vi "Module output.vi"   [LabVIEW 2015]
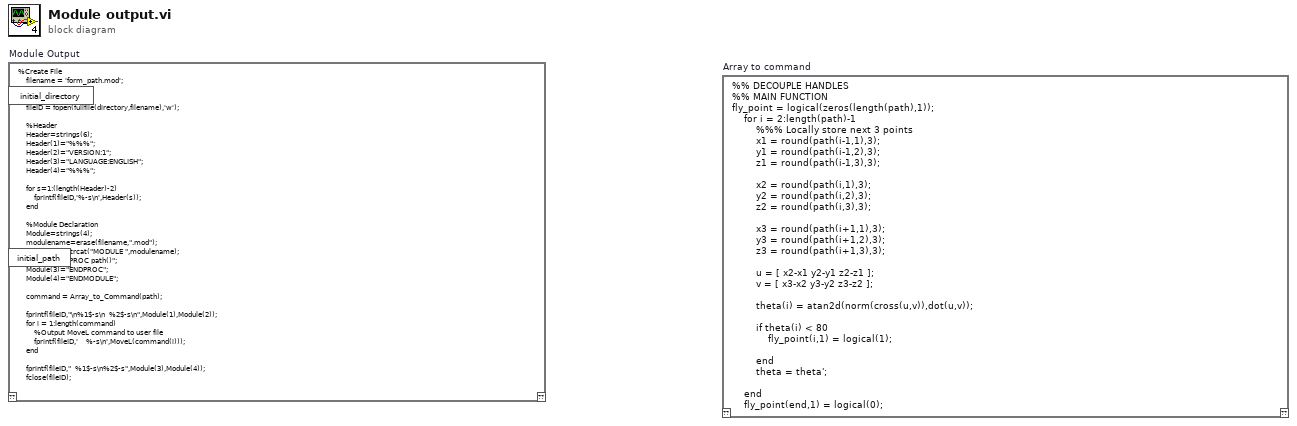
[diagram p0: block diagram]
diagram:
  n1 = script code="%Create File\n    filename = 'form_path.mod';\n   \n    %Open File\n    fileID = fopen(fullfile(directory,filename),'w');\n\n    %Header\n    Header=strings(6);\n    Header(1)=\"%%%\";\n    Header(2)=\"VERSION:1\";\n    Header(3)=\"LANGUAGE:ENGLISH\";\n    Header(4)=\"%%%\";\n    \n    for s=1:(length(Header)-2)\n        fprintf(fileID,'%-s\\n',Header(s));\n    end\n    \n    %Module Declaration\n    Module=strings(4);\n    modulename=erase(filename,\".mod\");\n    Module(1)=strcat(\"MODULE \",modulename);\n    Module(2)=\"PROC path()\";\n    Module(3)=\"ENDPROC\";\n    Module(4)=\"ENDMODULE\";\n    \n    command = Array_to_Command(path);\n    \n    fprintf(fileID,\"\\n%1$-s\\n  %2$-s\\n\",Module(1),Module(2));\n    for i = 1:length(command)\n        %Output MoveL command to user file\n        fprintf(fileID,'    %-s\\n',MoveL(command(i)));\n    end\n        \n    fprintf(fileID,\"  %1$-s\\n%2$-s\",Module(3),Module(4));\n    fclose(fileID);" "Module Output"() -> ()  [unwired: 3 in, 1 out]
  n2 = script code="%% DECOUPLE HANDLES\n%% MAIN FUNCTION\nfly_point = logical(zeros(length(path),1));\n    for i = 2:length(path)-1\n        %%% Locally store next 3 points\n        x1 = round(path(i-1,1),3);\n        y1 = round(path(i-1,2),3);\n        z1 = round(path(i-1,3),3);\n\n        x2 = round(path(i,1),3);\n        y2 = round(path(i,2),3);\n        z2 = round(path(i,3),3);\n\n        x3 = round(path(i+1,1),3);\n        y3 = round(path(i+1,2),3);\n        z3 = round(path(i+1,3),3);\n        \n        u = [ x2-x1 y2-y1 z2-z1 ];\n        v = [ x3-x2 y3-y2 z3-z2 ]; \n        \n        theta(i) = atan2d(norm(cross(u,v)),dot(u,v));\n        \n        if theta(i) < 80\n            fly_point(i,1) = logical(1);\n            \n        end\n        theta = theta';\n\n    end\n    fly_point(end,1) = logical(0);\n    \n    %%% Assign matrix to array of robtargets (command)\n    command = robtarget.empty(length(path),0);\n    for i = 1:length(path)\n        command(i,1).name = ['p',num2str(i)];\n        command(i,1).x = path(i,1);\n        command(i,1).y = path(i,2);\n        command(i,1).z = path(i,3);\n        if fly_point(i)\n            command(i,1).zone = 'z0';\n        end\n    end" "Array to command"() -> ()  [unwired: 1 in, 1 out]
